vi "Get Database.vi"(8 "error in (no error)":errorcluster, 11 "Table Configuration Adv Schema DB in":refnum<class "Table Configuration Adv Schema DB.lvclass">) -> (0 "error out":errorcluster, 2 "Database":refnum<class "Database Interface.lvclass">, 3 "Table Configuration Adv Schema DB out":refnum<class "Table Configuration Adv Schema DB.lvclass">)   [LabVIEW 2020, in "Table.lvlib" / "Table Configuration Adv Schema DB.lvclass"]
uses:
  Table Configuration Adv Schema DB.lvclass
  Database Libraries/Database Interfaces/Database Interface Class/Database Interface.lvclass
  Table Configuration Adv Schema DB.lvclass/Table Configuration Adv Schema DB.ctl
  Database Libraries/Database Interfaces/Database Advanced Schema Class/Database Adv Schema.lvclass
  C:/Users/User/Desktop/Raman Program/Database OOP/source/Database OOP/Database Libraries/Database Interfaces/Database Interface Class/Database Interface.lvclass
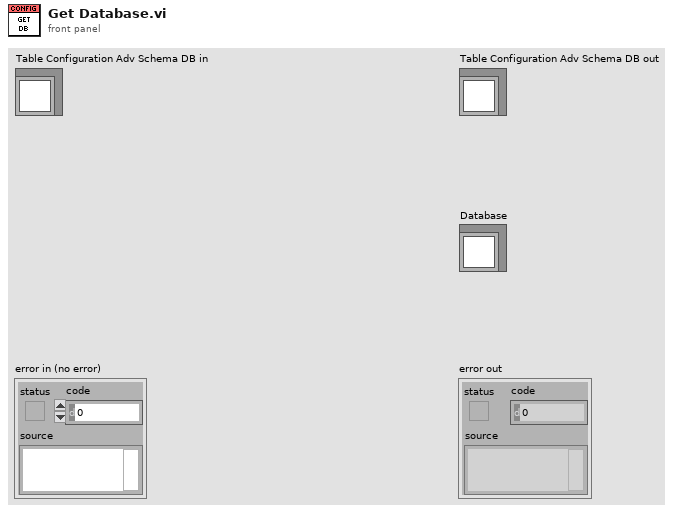
[diagram p1: front panel]
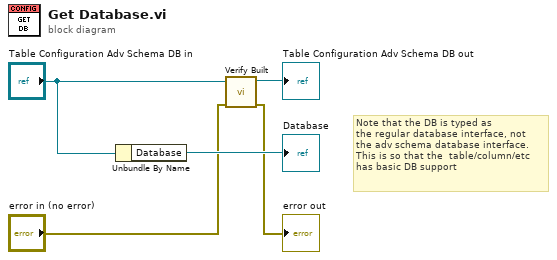
[diagram p0: block diagram]
diagram:
  # "Note that the DB is typed as\nthe regular database interface, not\nthe adv schema database interface.\nThis is so that the  table/column/etc\nhas basic DB support"
  n1 = Unbundle By Name("Table Configuration Adv Schema DB in") -> ("Database"=→"Database":refnum<class "Database Adv Schema.lvclass">)
  n2 = call-dynamic "Verify Built.vi"("error in (no error)"="error in (no error)", "Table Configuration in"="Table Configuration Adv Schema DB in") -> ("error out"=→"error out":errorcluster, "Table Configuration out"=→"Table Configuration Adv Schema DB out":refnum<class "Table Configuration Adv Schema DB.lvclass">)  [unwired: 8 in]
